vi "Run (SubVI).vi"(10 "MD5 message-digest":string, 11 "About_prg":T1) -> (3 "String":string)   [LabVIEW 2017]
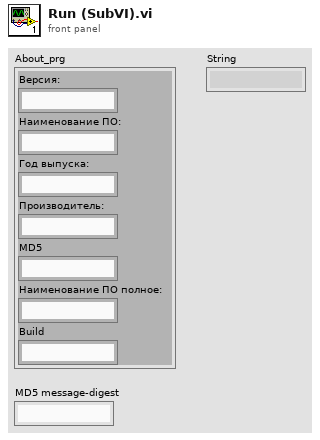
[diagram p1: front panel]
types:
  T1 = cluster{"Версия:":string, "Наименование ПО:":string, "Год выпуска:":string, "Производитель:":string, "MD5":string, "Наименование ПО полное:":string, "Build":string}
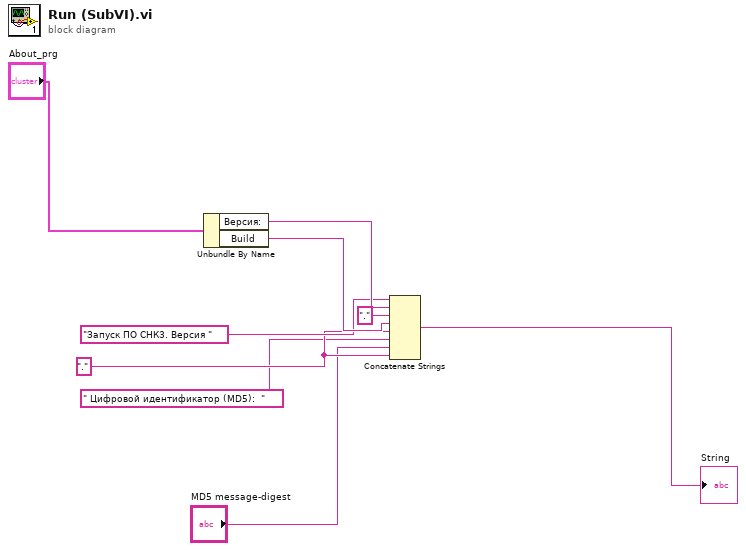
[diagram p0: block diagram]
diagram:
  w4 = "." ("string")
  n1 = Unbundle By Name("About_prg") -> ("Версия:"=w8:string, "Build"=w9:string)
  n2 = Concatenate Strings("Запуск ПО СНК3. Версия " ("string"), w8, "." ("string"), w9, w4, " Цифровой идентификатор (MD5):  " ("string"), "MD5 message-digest", w4) -> (→"String":string)
